vi "Add Routing and Faulting Custom Device.vi"(0 "Target in":refnum<k24>, 11 "error in (no error)":errorcluster) -> (4 "Target out":refnum<k24>, 6 "RAF Custom Device":refnum<k24>, 8 "Routes Section Ref":T1 format="%.0x", 10 "Aliases Section Ref":T1 format="%.0x", 15 "error out":errorcluster)   [LabVIEW 2017, in "Switch Scripting.lvlib"]
uses:
  Switch Scripting.lvlib
  NationalInstruments.VeriStand.SystemDefinitionAPI
  <vilib>/NI Veristand/Custom Device API/Custom Device Item Ref.ctl
  Shared/Constants.vi
  Shared/Switch Shared.lvlib
  <vilib>/NI VeriStand/Custom Device API/Custom Device API.lvlib
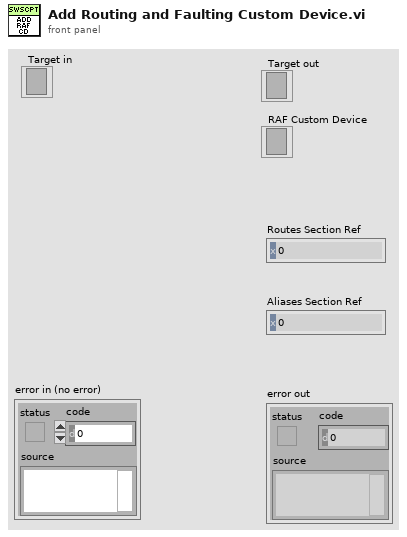
[diagram p1: front panel]
types:
  T1 = typedef "Custom Device API.lvlib/Custom Device Item Ref.ctl" = u64
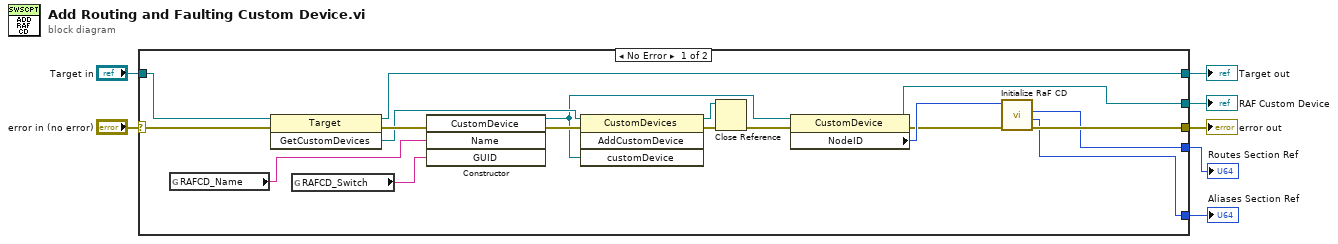
[diagram p0: block diagram]
diagram:
  n1 = case shown="No Error" "error in (no error)" {
    selector: "error in (no error)" -> [w25 w27]
    tunnel: [w11 w27] -> w7
    tunnel: "Target in" -> [w24 w26]
    tunnel: [w20 w26] -> w4
    tunnel: [w16 _] -> w3
    tunnel: [w10 _] -> w2
    tunnel: [w9 _] -> w1
    frame No Error {
      n2 = global read "Constants.vi" "RAFCD_Name"() -> (w8:string)
      n3 = invoke class="Target" method="GetCustomDevices"(reference=w24, error in=w25) -> (reference out=w20:refnum<k24>, error out=w23:errorcluster, "GetCustomDevices"=w22:refnum<k24>)  [unwired: 1 in]
      n4 = global read "Constants.vi" "RAFCD_Switch"() -> (w14:string)
      n5 = constructor class="CustomDevice"(error in=w23, "Name"=w8, "GUID"=w14) -> (reference out=w17:refnum<k24>, error out=w21:errorcluster)  [unwired: 2 in, 3 out]
      n6 = invoke class="CustomDevices" method="AddCustomDevice"(reference=w22, error in=w21, "customDevice"=w17) -> (reference out=w19:refnum<k24>, error out=w18:errorcluster)  [unwired: 1 in, 2 out]
      n7 = Close Reference(reference=w19, error in (no error)=w18) -> (error out=w15:errorcluster)
      n8 = property class="CustomDevice"(reference=w17, error in=w15) -> (reference out=w16:refnum<k24>, error out=w12:errorcluster, "NodeID"=w13:u64)
      n9 = call "Initialize RaF CD.vi"("error in (no error)"=w12, "RaF CD Ref in"=w13) -> ("error out"=w11:errorcluster, "Aliases Section Ref"=w9:T1, "Routes Section Ref"=w10:T1)  [unwired: 6 in, 1 out]
    }
    frame Error {
    }
  }
  "Target out" <- w4
  "error out" <- w7
  "RAF Custom Device" <- w3
  "Routes Section Ref" <- w2
  "Aliases Section Ref" <- w1
